vi "Create Transfer Group Configuration.vi"(6 "group timing (dec:1, off: 0)":T6={"priority"=0, "decimation"=1, "offset"=0}, 7 "base group name (group)":string="group", 8 "settings":T1, 9 "direction":T5, 11 "transfer configs":T3(array[cluster])) -> (3 "Transfer Group":T4={"name"="", "direction"=enum."Tx", "cycle timing"={"priority"=0, "decimation"=1, "offset"=0}, "Transfers"=[], "settings"=[]} {"Transfers"."channel configurations"."buffer offset" format="%d bytes"})   [LabVIEW 2017]
uses:
  Builds/Data Sharing Framework/Current/Data Sharing Framework Core/DSF Core.lvlibp/Configuration/Public/Controls/DSF Timing Info.ctl
  Builds/Data Sharing Framework/Current/Data Sharing Framework Core/DSF Core.lvlibp/Configuration/Public/Controls/DSF Direction.ctl
  Builds/Data Sharing Framework/Current/Data Sharing Framework Core/DSF Core.lvlibp/Configuration/Public/Controls/DSF Engine Transfer Group Configuration.ctl
  Builds/Data Sharing Framework/Current/Data Sharing Framework Core/DSF Core.lvlibp/Configuration/Public/Controls/DSF Engine Transfer Configuration.ctl
  Builds/Data Sharing Framework/Current/Data Sharing Framework Core/DSF Core.lvlibp/Configuration/Public/Controls/DSF Byte Order.ctl
  Builds/Data Sharing Framework/Current/Data Sharing Framework Core/DSF Core.lvlibp/Configuration/Public/Controls/DSF Engine Channel Configuration.ctl
  Builds/Data Sharing Framework/Current/Data Sharing Framework Core/DSF Core.lvlibp/Configuration/Public/Controls/DSF Data Type.ctl
  Builds/Data Sharing Framework/Current/Data Sharing Framework Core/DSF Core.lvlibp/Configuration/Public/Controls/DSF Settings Info.ctl
  Builds/Data Sharing Framework/Current/Data Sharing Framework Core/DSF Core.lvlibp
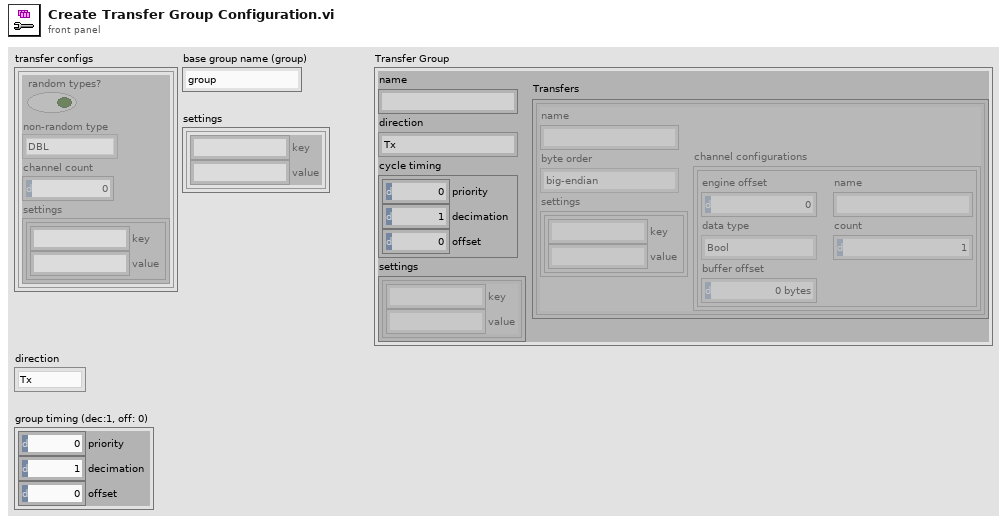
[diagram p1: front panel]
types:
  T1 = typedef "DSF Core.lvlibp/DSF Settings Info.ctl" = cluster{"key":string, "value":string}[]
  T2 = typedef "DSF Core.lvlibp/DSF Data Type.ctl" = enum8{"Bool", "SGL", "DBL", "I8", "I16", "I32", "I64", "U8", "U16", "U32", "U64"}
  T3 = cluster{"random types?":bool, "non-random type":T2, "channel count":i32, "settings":T1}[]
  T4 = typedef "DSF Core.lvlibp/DSF Engine Transfer Group Configuration.ctl" = cluster{"name":string, "direction":T5, "cycle timing":T6, "Transfers":T7[], "settings":T1}
  T5 = typedef "DSF Core.lvlibp/DSF Direction.ctl" = enum8{"Tx", "Rx"}
  T6 = typedef "DSF Core.lvlibp/DSF Timing Info.ctl" = cluster{"priority":u64, "decimation":u64, "offset":u64}
  T7 = typedef "DSF Core.lvlibp/DSF Engine Transfer Configuration.ctl" = cluster{"name":string, "byte order":T8, "channel configurations":T9[], "settings":T1}
  T8 = typedef "DSF Core.lvlibp/DSF Byte Order.ctl" = enum8{"big-endian", "little-endian"}
  T9 = typedef "DSF Core.lvlibp/DSF Engine Channel Configuration.ctl" = cluster{"engine offset":u64, "name":string, "data type":T2, "count":u64, "buffer offset":u64}
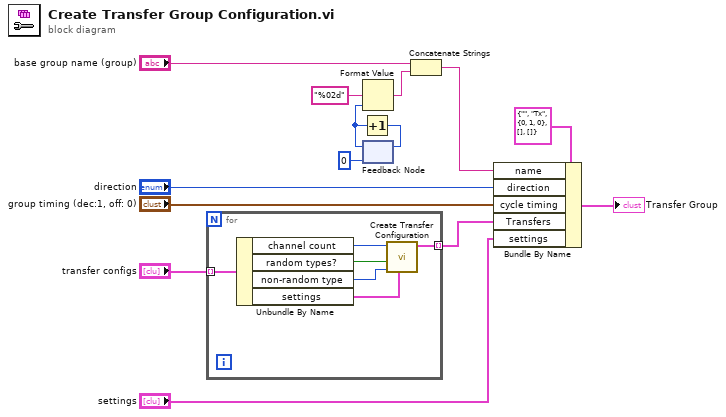
[diagram p0: block diagram]
diagram:
  n1 = for {
    tunnel: [w20] -> w3 mode=indexing
    tunnel: "transfer configs" -> [w19] mode=indexing
    n2 = Unbundle By Name(w19) -> ("channel count"=w16:i32, "random types?"=w15:bool, "non-random type"=w18:T2, "settings"=w17:T1)
    n3 = call "Create Transfer Configuration.vi"("settings"=w17, "non-random type (DBL)"=w18, "random types? (F)"=w15, "channel count"=w16) -> ("Transfers"=w20:T7)  [unwired: 7 in]
  }
  n4 = feedback #1(0) -> (w13:i32)
  n5 = Increment(x=w13) -> (x+1=w11:i32)
  n6 = Format Value(format string="%02d", value (0)=w13) -> (output string=w8:string)  [unwired: 1 in]
  n7 = feedback-in #1(w11) -> ()
  n8 = Concatenate Strings("base group name (group)", w8) -> (w2:string)
  n9 = Bundle By Name(cluster=T4 {"name"="", "direction"=enum."Tx", "cycle timing"={"priority"=0, "decimation"=1, "offset"=0}, "Transfers"=[], "settings"=[]} ("Transfer Groups"), "name"=w2, "direction"="direction", "cycle timing"="group timing (dec:1, off: 0)", "Transfers"=w3, "settings"="settings") -> (→"Transfer Group":T4)
